vi "Sequence.CreateMonitorVariable.vi"(7 "Iteration":string, 8 "error in (no error)":errorcluster, 10 "StepInfo":T1, 11 "Task Ref":refnum<k24>) -> (0 "error out":errorcluster, 3 "Task Ref out":refnum<k24>)   [LabVIEW 2013, in "Simple Sequence Tools - Editor.lvlib"]
uses:
  Simple Sequence Tools - Editor.lvlib
  Shared/Types/ChannelProperties.ctl
  NationalInstruments.VeriStand.RealTimeSequenceDefinitionApi
  Shared/Simple Sequence Tools - Shared.lvlib
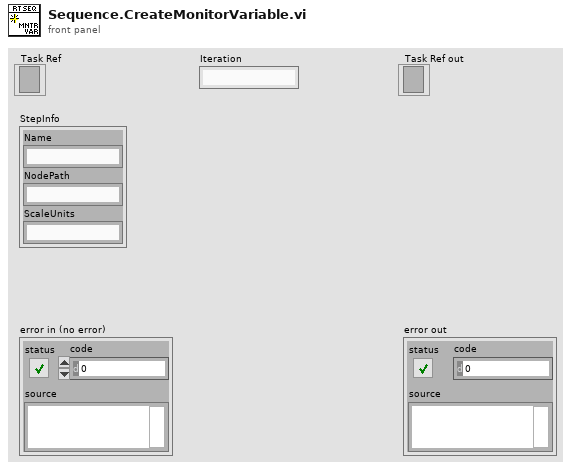
[diagram p1: front panel]
types:
  T1 = typedef "Simple Sequence Tools - Shared.lvlib/ChannelProperties.ctl" = cluster{"Name":string, "NodePath":string, "ScaleUnits":string}
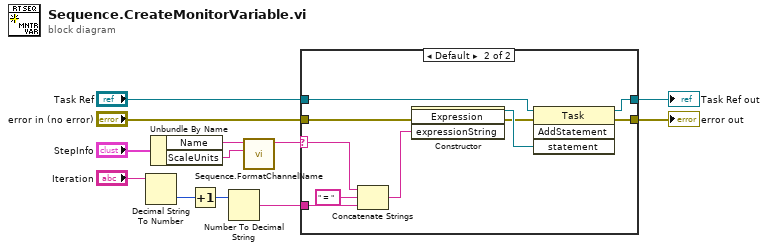
[diagram p0: block diagram]
diagram:
  n1 = Decimal String To Number(string="Iteration") -> (number=w3:i32)  [unwired: 2 in, 1 out]
  n2 = Unbundle By Name("StepInfo") -> ("Name"=w9:string, "ScaleUnits"=w10:string)
  n3 = Increment(x=w3) -> (x+1=w2:i32)
  n4 = Number To Decimal String(number=w2) -> (decimal integer string=w1:string)  [unwired: 1 in]
  n5 = call "Sequence.FormatChannelName.vi"("ScaleUnits"=w10, "Name"=w9) -> ("ChannelName"=w12:string)  [unwired: 9 in]
  n6 = case shown="Default" w12 {
    selector: w12 -> [_ w16]
    tunnel: [w14 w24] -> w5
    tunnel: "Task Ref" -> [w13 w23]
    tunnel: [w13 w22] -> w4
    tunnel: "error in (no error)" -> [w14 w18]
    tunnel: w1 -> [_ w15]
    frame "" {
    }
    frame Default {
      n7 = Concatenate Strings(w16, " = " ("string"), w15) -> (w20:string)
      n8 = constructor class="Expression"(error in=w18, "expressionString"=w20) -> (reference out=w19:refnum<k24>, error out=w17:errorcluster)  [unwired: 2 in, 2 out]
      n9 = invoke class="Task" method="AddStatement"(reference=w23, error in=w17, "statement"=w19) -> (reference out=w22:refnum<k24>, error out=w24:errorcluster)  [unwired: 1 in, 2 out]
    }
  }
  "error out" <- w5
  "Task Ref out" <- w4
